vi "Load Color Selector.vi"(8 "error in (no error)":errorcluster, 10 "Grey Scale Index (0-255)":u8, 11 "ColorSelector in":refnum<class "ColorSelector.lvclass">) -> (0 "error out":errorcluster, 3 "ColorSelector out":refnum<class "ColorSelector.lvclass">)   [LabVIEW 2020, in "ColorSelector.lvclass"]
doc: "This VI draws the Color Selector based on the Hue Array and the selected Grey from the Grey Selector.\n<b> </b> <b> </b>\n©2017 Q Software Innovations, LLC (QSI)\nwritten by Quentin Alldredge\nproduced in LabVIEW 2015\n\nsupport@qsoftwareinnovations.com\nwww.qsoftwareinnovations.com\n\nAll rights reserved.\n\nRedistribution and use in source and binary forms, with or without modification, are permitted provided that the following conditions are met:\n\n * Redistributions of source code must retain the above copyright notice, this list of conditions and the following disclaimer.\n * Redistributions in binary form must reproduce the above copyright notice, this list of conditions and the following disclaimer in the documentation and/or other materials provided with the distribution.\n * Neither the name of Q Software Innovations, LLC. nor the names of its contributors may be used to endorse or promote products derived from this software without specific prior written permission.\n\nTHIS SOFTWARE IS PROVIDED BY THE COPYRIGHT HOLDERS AND CONTRIBUTORS \"AS IS\" AND ANY EXPRESS OR IMPLIED WARRANTIES, INCLUDING, BUT NOT LIMITED TO, THE IMPLIED WARRANTIES OF MERCHANTABILITY AND FITNESS FOR A PARTICULAR PURPOSE ARE DISCLAIMED. IN NO EVENT SHALL THE COPYRIGHT OWNER OR CONTRIBUTORS BE LIABLE FOR ANY DIRECT, INDIRECT, INCIDENTAL, SPECIAL, EXEMPLARY, OR CONSEQUENTIAL DAMAGES (INCLUDING, BUT NOT LIMITED TO, PROCUREMENT OF SUBSTITUTE GOODS OR SERVICES; LOSS OF USE, DATA, OR PROFITS; OR BUSINESS INTERRUPTION) HOWEVER CAUSED AND ON ANY THEORY OF LIABILITY, WHETHER IN CONTRACT, STRICT LIABILITY, OR TORT (INCLUDING NEGLIGENCE OR OTHERWISE) ARISING IN ANY WAY OUT OF THE USE OF THIS SOFTWARE, EVEN IF ADVISED OF THE POSSIBILITY OF SUCH DAMAGE."
uses:
  ColorSelector.lvclass
  <vilib>/picture/picture.llb/imagedata.ctl
  ColorSelector.lvclass/ColorSelector.ctl
  Read Hue[].vi
  Write ColorSelectPic.vi
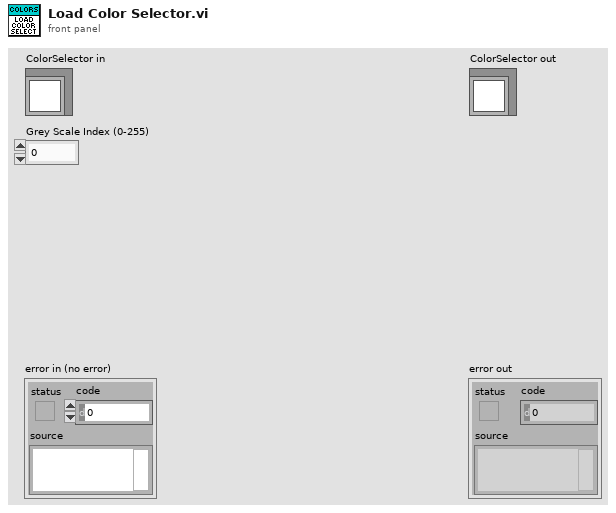
[diagram p1: front panel]
types:
  T1 = typedef "imagedata.ctl" = cluster{"image type":i32, "image depth":i32, "image":u8[], "mask":u8[], "colors":u32[], "Rectangle":cluster{"left":i16, "top":i16, "right":i16, "bottom":i16}}
  T2 = typedef "LVBoundsTypeDef.ctl" = cluster{"Width":u32, "Height":u32}
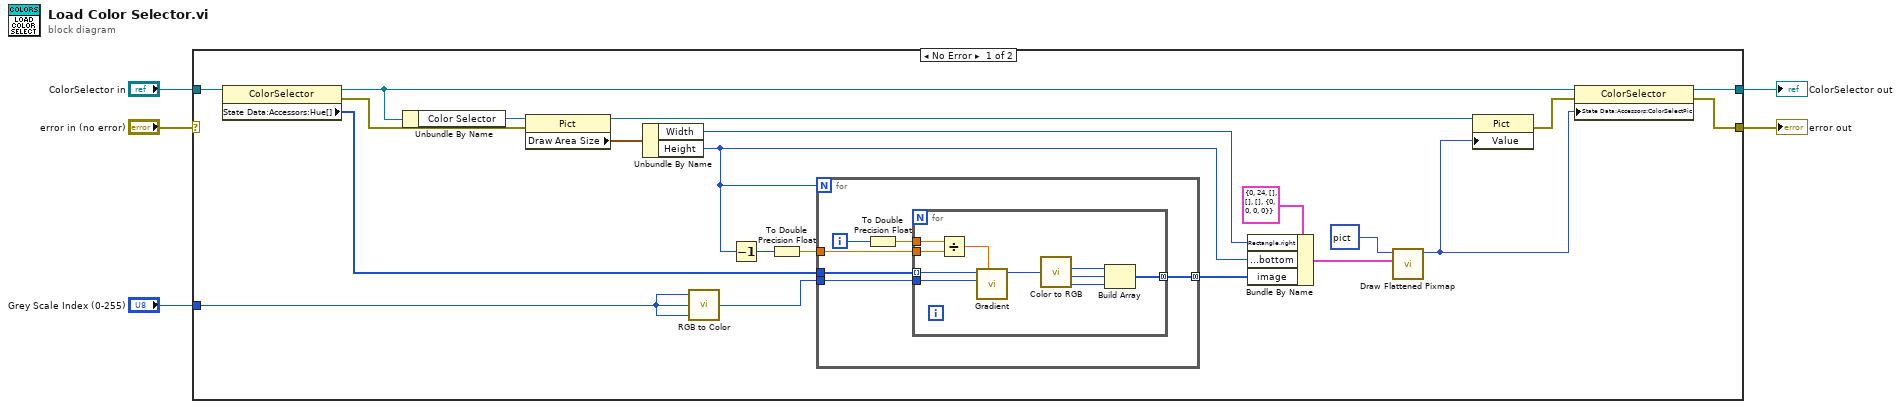
[diagram p0: block diagram]
diagram:
  n1 = case shown="No Error" "error in (no error)" {
    selector: "error in (no error)" -> [_ w43]
    tunnel: "ColorSelector in" -> [w18 w44]
    tunnel: [w14 w44] -> w3
    tunnel: "Grey Scale Index (0-255)" -> [w9 _]
    tunnel: [w11 w43] -> w1
    frame No Error {
      n2 = property class="ColorSelector"(reference=w18) -> (reference out=w17:refnum<class "ColorSelector.lvclass">, error out=w15:errorcluster, "State Data:Accessors:Hue[]"=w16:u32[])  [unwired: 1 in]
      n3 = Unbundle By Name(w17) -> ("Color Selector"=w26:refnum<vi>)
      n4 = property class="Pict"(reference=w26, error in=w15) -> (reference out=w24:refnum<vi>, "Draw Area Size"=w25:T2)  [unwired: 1 out]
      n5 = Unbundle By Name(w25) -> ("Width"=w19:u32, "Height"=w10:u32)
      n6 = call <vilib>:"RGB to Color.vi"("B"=w9, "G"=w9, "R"=w9) -> ("Color"=w8:u32)
      n7 = Decrement(x=w10) -> (x-1=w7:u32)
      n8 = To Double Precision Float(number=w7) -> (double precision float=w6:dbl)
      n9 = for {
        N: w10 -> [_]
        tunnel: w16 -> [w32]
        tunnel: w8 -> [w31]
        tunnel: [w30] -> w20 mode=concatenating
        tunnel: w6 -> [w27]
        i -> [w29]
        n10 = To Double Precision Float(number=w29) -> (double precision float=w28:dbl)
        n11 = for {
          tunnel: w32 -> [w42] mode=indexing
          tunnel: w31 -> [w41]
          tunnel: w28 -> [w34]
          tunnel: w27 -> [w40]
          tunnel: [w36] -> w30 mode=concatenating
          n12 = Divide(x=w34, y=w40) -> (x/y=w33:dbl)
          n13 = call "Gradient.vi"("Percent"=w33, "End Color"=w41, "Start Color"=w42) -> ("Gradient Color"=w35:u32)  [unwired: 8 in]
          n14 = call <vilib>:"Color to RGB.vi"("Color"=w35) -> ("R"=w39:u8, "G"=w38:u8, "B"=w37:u8)  [unwired: 1 out]
          n15 = Build Array(w39, w38, w37) -> (w36:u8[])
        }
      }
      n16 = Bundle By Name(cluster=T1 {"image type"=0, "image depth"=24, "image"=[], "mask"=[], "colors"=[], "Rectangle"={"left"=0, "top"=0, "right"=0, "bottom"=0}} ("image data"), "Rectangle.right"=w19, "Rectangle.bottom"=w10, "image"=w20) -> (w23:T1)
      n17 = call <vilib>:"Draw Flattened Pixmap.vi"("image data"=w23, "picture"=picture data[5B] ("new picture")) -> ("new picture"=w13:picture)  [unwired: 7 in]
      n18 = property class="Pict"(reference=w24, "Value"=w13) -> (error out=w12:errorcluster)  [unwired: 1 in, 1 out]
      n19 = property class="ColorSelector"(reference=w17, error in=w12, "State Data:Accessors:ColorSelectPic"=w13) -> (reference out=w14:refnum<class "ColorSelector.lvclass">, error out=w11:errorcluster)
    }
    frame Error {
    }
  }
  "error out" <- w1
  "ColorSelector out" <- w3
